vi "Initialize.vi"(8 "error in (no error)":errorcluster, 11 "State in":T1={"State"=enum."Idle", "Start Time"=timestamp(0 s since 1904-01-01), "Configuration"={"Cycle Period"=0.0, "Mettler"={"VISA resource name"="", "Simulated?"=FALSE}, "Scale Type"=""}, "Current Time"=timestamp(0 s since 1904-01-01), "First Iteration"=FALSE, "Data"={"Scale Read(g)"=0.0}, "Process Name"="", "Log Started"=FALSE}) -> (0 "error out":errorcluster, 3 "State out":T1={"State"=enum."Idle", "Start Time"=timestamp(0 s since 1904-01-01), "Configuration"={"Cycle Period"=0.0, "Mettler"={"VISA resource name"="", "Simulated?"=FALSE}, "Scale Type"=""}, "Current Time"=timestamp(0 s since 1904-01-01), "First Iteration"=FALSE, "Data"={"Scale Read(g)"=0.0}, "Process Name"="", "Log Started"=FALSE})   [LabVIEW 2018, in "Sonicator Module.lvlib" / "Sonicator Module Engine.lvlib"]
uses:
  Sonicator Module Engine.lvlib
  State Cluster.ctl
  State Enum.ctl
  Feed Module/Controls/Sonicator Module Settings Cluster.ctl
  Mettler Toledo/Controls/Settings Cluster.ctl
  Tag VIs/Tag FGV Operation Enum.ctl
  Mettler Toledo/Mettler Toledo.lvlib
  Shared Variables/Dynamic Shared Variables.lvlib
  Sonicator Module.lvlib
panel:
  # "Scale Settings"
  # "Scale Settings"
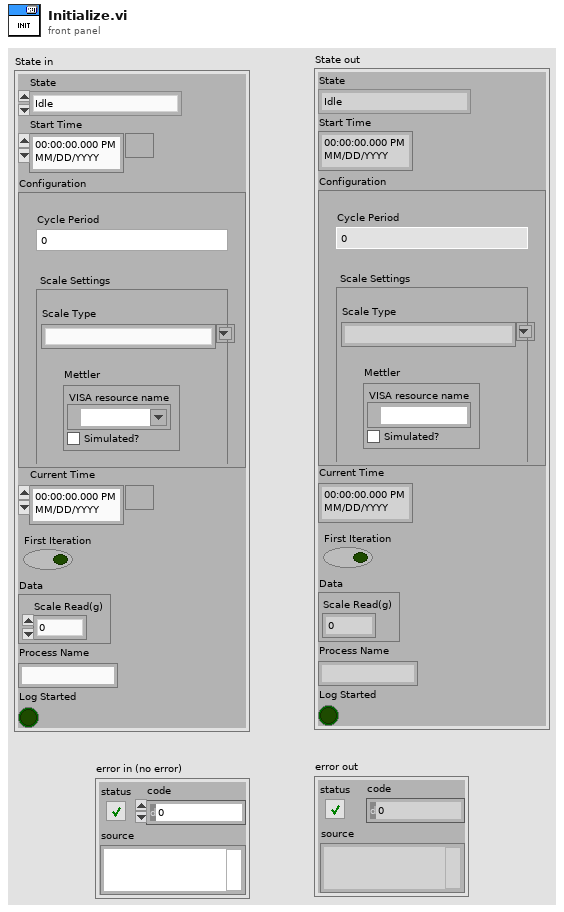
[diagram p1: front panel]
types:
  T1 = typedef "Sonicator Module.lvlib/Sonicator Module Engine.lvlib/State Cluster.ctl" = cluster{"State":T2, "Start Time":timestamp, "Configuration":T3, "Current Time":timestamp, "First Iteration":bool, "Data":cluster{"Scale Read(g)":dbl}, "Process Name":string, "Log Started":bool}
  T2 = typedef "Sonicator Module.lvlib/Sonicator Module Engine.lvlib/State Enum.ctl" = enum16{"Measuring", "Idle"}
  T3 = typedef "Sonicator Module.lvlib/Sonicator Module Settings Cluster.ctl" = cluster{"Cycle Period":dbl, "Mettler":T4, "Scale Type":string}
  T4 = typedef "Mettler Toledo.lvlib/Settings Cluster.ctl" = cluster{"VISA resource name":refnum<visa-resource-name>, "Simulated?":bool}
  T5 = typedef "Tag FGV Operation Enum.ctl" = enum16{"Init", "Set Notification Queue", "Create Tag", "Commit", "Write Tag (Numeric)", "Write Tag (Boolean)", "Read All Tags", "Read One Tag", "Delete Tag Category", "Set Alarm Parameters (Numeric)", "Set Alarm Parameters (Boolean)", "Enable All Alarms", "Disable All Alarms", "Delete All Tags", "Read Alarms", "Ack Alarm", "Read Alarm Parameters (Numeric)", "Read Alarm Parameters (Boolean)"}
  T6 = cluster{"Scale Tag":string, "Output Device Tag":string}
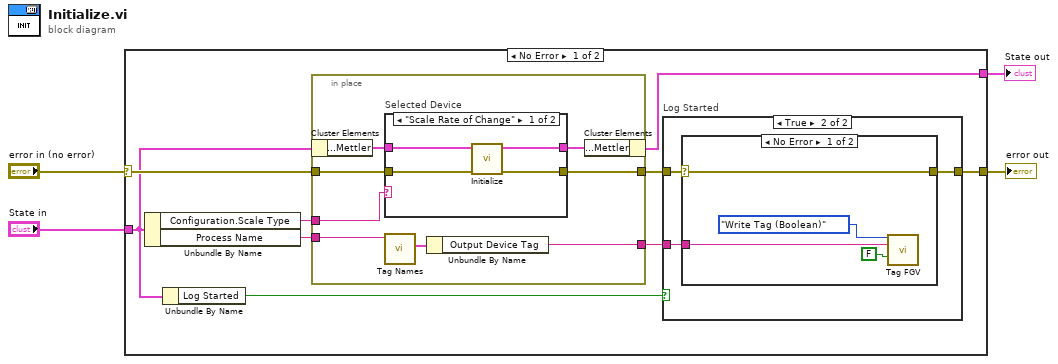
[diagram p0: block diagram]
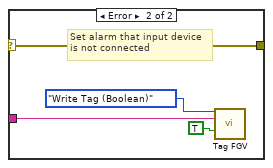
[diagram p4: hidden frame]
diagram:
  n1 = case shown="No Error" "error in (no error)" {
    selector: "error in (no error)" -> [w12 w41]
    tunnel: [w9 w41] -> w3
    tunnel: "State in" -> [w6 w40]
    tunnel: [w5 w40] -> w1
    frame No Error {
      n2 = Unbundle By Name(w6) -> ("Configuration.Scale Type"=w13:string, "Process Name"=w11:string)
      n3 = Unbundle By Name(w6) -> ("Log Started"=w7:bool)
      n4 = in-place {
        in-place-border: w13 -> [w21]
        in-place-border: w12 -> [w20]
        in-place-border: w11 -> [w19]
        in-place-border: [w18] -> w10
        in-place-border: [w16] -> w8
        n5 = in-place-cluster #1(w6) -> ("Configuration.Mettler"=w15:T4)
        n6 = case "Selected Device" shown="\"Scale Rate of Change\"" w21 {
          tunnel: w15 -> [w23 w27]
          tunnel: w20 -> [w22 w26]
          tunnel: [w24 w26] -> w18
          tunnel: [w25 w27] -> w14
          frame "Scale Rate of Change" {
            n7 = call "Initialize.vi"("error in (no error)"=w22, "Mettler Settings in"=w23) -> ("error out"=w24:errorcluster, "Mettler Settings out"=w25:T4)  [unwired: 7 in, 1 out]
          }
          frame "Default", Default {
          }
        }
        n8 = call "Tag Names.vi"("Process Name"=w19) -> ("Scale Tags"=w17:T6)  [unwired: 8 in, 2 out]
        n9 = Unbundle By Name(w17) -> ("Output Device Tag"=w16:string)
        n10 = in-place-cluster #1("Configuration.Mettler"=w14) -> (w5:T1)
      }
      n11 = case "Log Started" shown="True" w7 {
        tunnel: w10 -> [w28 w31]
        tunnel: [w28 w30] -> w9
        tunnel: w8 -> [_ w29]
        frame False {
        }
        frame True {
          n12 = case shown="No Error" w31 {
            selector: w31 -> [w35 w39]
            tunnel: [w35 w39] -> w30
            tunnel: w29 -> [w33 w37]
            frame No Error {
              n13 = call "Tag FGV.vi"("Operation"=Tag_FGV_Operation_Enum."Write Tag (Boolean)", "Tag Name"=w33, "Data"=FALSE) -> ()  [unwired: 5 in, 8 out]
            }
            frame Error {
              # "Set alarm that input device\nis not connected"
              n14 = call "Tag FGV.vi"("Operation"=Tag_FGV_Operation_Enum."Write Tag (Boolean)", "Tag Name"=w37, "Data"=TRUE) -> ()  [unwired: 5 in, 8 out]
            }
          }
        }
      }
    }
    frame Error {
    }
  }
  "error out" <- w3
  "State out" <- w1
